vi "PerformMeasurement.vi"(8 "error in (no error)":errorcluster, 10 "gRPCid":T4, 11 "ctet_smu":T1) -> (0 "error out":errorcluster, 3 "ctet_smu out":T1)   [LabVIEW 2019, in "ctet_smu User Library.lvlib"]
uses:
  ctet_smu User Library.lvlib
  Servers/ctet_smu/gRPC lvSupport/Server API/typeDefs/grpcId.ctl
  Types/ctet_smu.ctl
  Servers/ctet_smu/ctet_smu Class/RPC Messages/measurementservice_SMUConfigResponse/measurementservice_SMUConfigResponse_Data.ctl
  Servers/ctet_smu/ctet_smu Class/RPC Messages/measurementservice_ErrorOut/measurementservice_ErrorOut_Data.ctl
  Servers/ctet_smu/ctet_smu Class/RPC Messages/measurementservice_SMUCurrentData/measurementservice_SMUCurrentData_Data.ctl
  Servers/ctet_smu/ctet_smu Class/ctet_smu.lvclass
  Servers/ctet_smu/gRPC lvSupport/gprc-lvsupport.lvlib
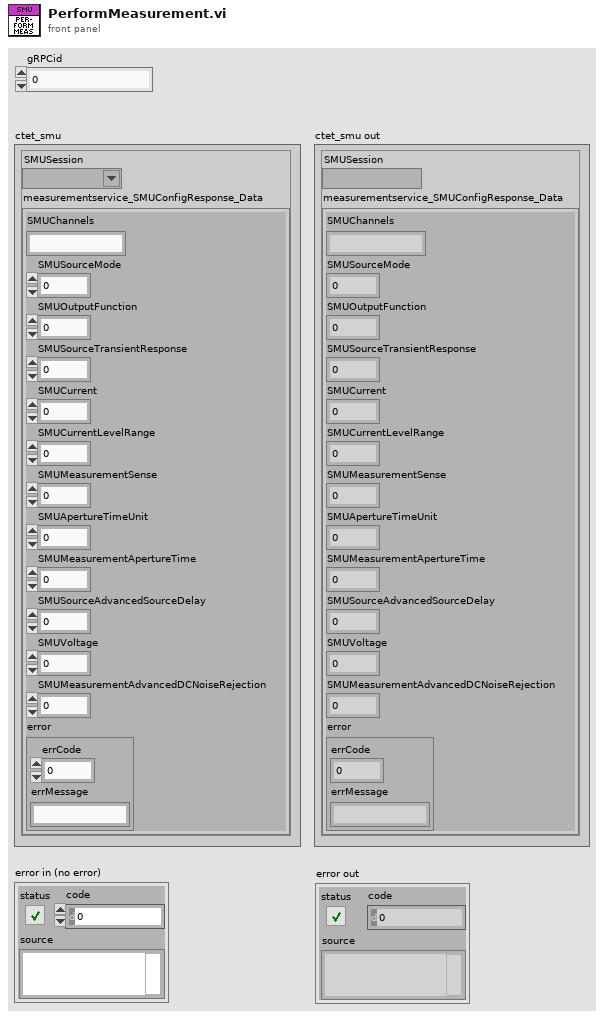
[diagram p1: front panel]
types:
  T1 = typedef "ctet_smu User Library.lvlib/ctet_smu.ctl" = cluster{"SMUSession":refnum<k15>, "measurementservice_SMUConfigResponse_Data":T2}
  T2 = typedef "ctet_smu.lvlib/ctet_smu.lvclass/measurementservice_SMUConfigResponse_Data.ctl" = cluster{"SMUChannels":string, "SMUSourceMode":i64, "SMUOutputFunction":i64, "SMUSourceTransientResponse":i64, "SMUCurrent":dbl, "SMUCurrentLevelRange":dbl, "SMUMeasurementSense":i64, "SMUApertureTimeUnit":i64, "SMUMeasurementApertureTime":dbl, "SMUSourceAdvancedSourceDelay":dbl, "SMUVoltage":dbl, "SMUMeasurementAdvancedDCNoiseRejection":i64, "error":T3}
  T3 = typedef "ctet_smu.lvlib/ctet_smu.lvclass/measurementservice_ErrorOut_Data.ctl" = cluster{"errCode":i64, "errMessage":string}
  T4 = typedef "ctet_smu.lvlib/gprc-lvsupport.lvlib/grpcId.ctl" = u64
  T5 = typedef "ctet_smu.lvlib/ctet_smu.lvclass/measurementservice_SMUCurrentData_Data.ctl" = cluster{"current":dbl, "error":T3}
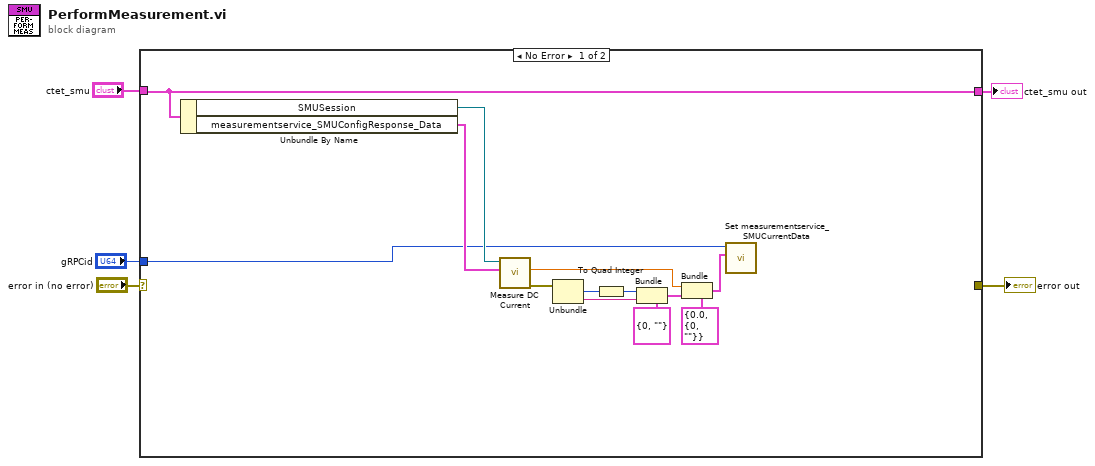
[diagram p0: block diagram]
diagram:
  n1 = case shown="No Error" "error in (no error)" {
    selector: "error in (no error)" -> [_ w20]
    tunnel: [_ w20] -> w5
    tunnel: "gRPCid" -> [w15 _]
    tunnel: "ctet_smu" -> [w16 w19]
    tunnel: [w16 w19] -> w1
    frame No Error {
      n2 = Unbundle By Name(w16) -> ("SMUSession"=w18:refnum<k15>, "measurementservice_SMUConfigResponse_Data"=w17:T2)
      n3 = call "Measure DC Current.vi"("measurementservice_SMUConfigResponse_Data"=w17, "SMUSession"=w18) -> ("error out"=w12:errorcluster, "Current Measurement"=w9:dbl)  [unwired: 6 in, 2 out]
      n4 = Unbundle(w12) -> ("code"=w7:i32, "source"=w8:string)  [unwired: 1 out]
      n5 = To Quad Integer(1:w7) -> (0:w6:i64)
      n6 = Bundle(cluster=T3 {"errCode"=0, "errMessage"=""} ("error"), "errCode"=w6, "errMessage"=w8) -> (w10:T3)
      n7 = Bundle(cluster=T5 {"current"=0.0, "error"={"errCode"=0, "errMessage"=""}} ("Message Data"), "current"=w9, "error"=w10) -> (w13:T5)
      n8 = call "Set measurementservice_SMUCurrentData.vi"("Message Data"=w13, "gRPCid"=w15) -> ()  [unwired: 9 in, 1 out]
    }
    frame Error {
    }
  }
  "error out" <- w5
  "ctet_smu out" <- w1
